vi "optogeneticsTarget3D.vi"(1 "z mode":u16(ring) items=["optogenetics space", "imaging space"], 2 "z device":u16(ring) items=["etl", "piezo"], 3 "xy mode":u16(ring) items=["galvo space", "camera space"], 4 "xyz":dbl[](array[numeric])=[0.0, 0.0, 0.0]) -> ()   [LabVIEW 2017]
uses:
  globalUtilities.vi
  <vilib>/Analysis/NI_AALPro.lvlib
  <vilib>/Analysis/polynomials.llb/Scalar Polynomial Evaluation (DBL).vi
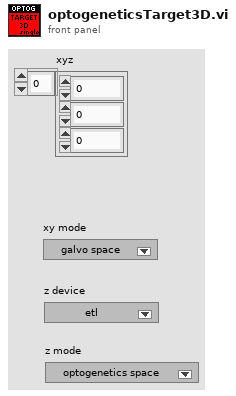
[diagram p1: front panel]
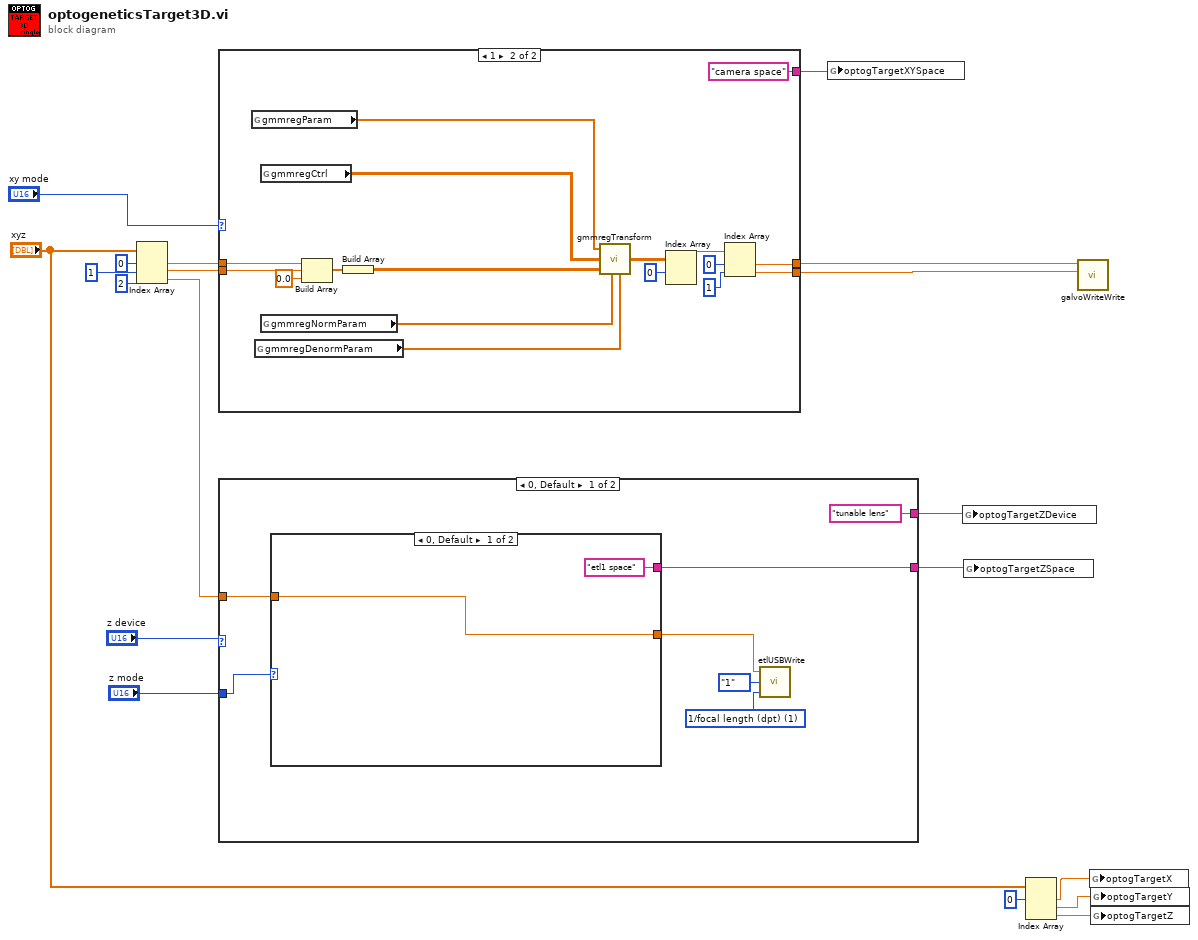
[diagram p0: block diagram]
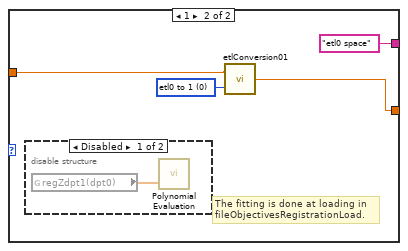
[diagram p2: hidden frame]
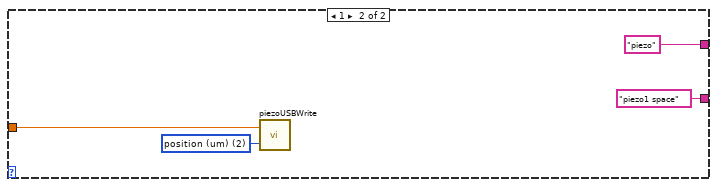
[diagram p4: hidden frame]
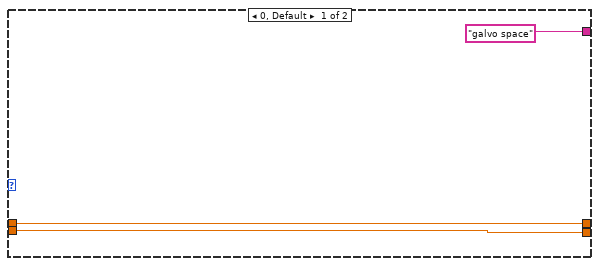
[diagram p5: hidden frame]
diagram:
  n1 = Index Array(array="xyz", index #1=0 ("index"), index #2=1 ("index"), index #3=2 ("index")) -> (element #1=w16:dbl, element #2=w15:dbl, element #3=w10:dbl)
  n2 = case shown="1" "xy mode" {
    tunnel: w16 -> [w22 w36]
    tunnel: w15 -> [w21 w35]
    tunnel: [w22 w26] -> w13
    tunnel: [w21 w25] -> w12
    tunnel: ["galvo space" "camera space"] -> w3
    frame 0, Default {
    }
    frame 1 {
      n3 = global read "globalUtilities.vi" "gmmregParam"() -> (w24:dbl[])
      n4 = global read "globalUtilities.vi" "gmmregDenormParam"() -> (w37:dbl[])
      n5 = global read "globalUtilities.vi" "gmmregCtrl"() -> (w39:dbl[][])
      n6 = global read "globalUtilities.vi" "gmmregNormParam"() -> (w38:dbl[])
      n7 = Build Array(w36, w35, 0.0 ("element")) -> (w33:dbl[])
      n8 = Build Array(w33) -> (w32:dbl[][])
      n9 = call "gmmregTransform.vi"("param0"=w24, "ctrlPts"=w39, "pts"=w32, "normParams"=w38, "denormParams"=w37) -> ("out"=w31:dbl[][])  [unwired: 4 in]
      n10 = Index Array(array=w31, index (row)=0) -> (element=w29:dbl[])  [unwired: 1 in]
      n11 = Index Array(array=w29, index #1=0 ("index"), index #2=1 ("index")) -> (element #1=w26:dbl, element #2=w25:dbl)
    }
  }
  n12 = case shown="0, Default" "z device" {
    tunnel: w10 -> [w45 w57]
    tunnel: "z mode" -> [w46 _]
    tunnel: ["tunable lens" "piezo"] -> w1
    tunnel: [w40 "piezo1 space"] -> w2
    frame 0, Default {
      w43 = u16 1 items=["position (um)", "1/focal length (dpt)"] ("mode")
      n13 = case shown="0, Default" w46 {
        tunnel: w45 -> [w48 w52]
        tunnel: [w48 w50] -> w42
        tunnel: ["etl1 space" "etl0 space"] -> w40
        frame 0, Default {
        }
        frame 1 {
          w51 = u16 0 items=["etl0 to 1", "etl1 to 0"] ("mode")
          # "The fitting is done at loading in\nfileObjectivesRegistrationLoad."
          n14 = disable-structure shown="Disabled" {
            frame Disabled {
              n15 = global read "globalUtilities.vi" "regZdpt1(dpt0)"() -> (w53:dbl[])
              n16 = call-poly <vilib>:"Polynomial Evaluation.vi"("P(x)"=w53) -> ()  [unwired: 1 in, 2 out]
            }
            frame Enabled {
            }
          }
          n17 = call "etlConversion01.vi"("mode"=w51, "in"=w52) -> ("out"=w50:dbl)
        }
      }
      n18 = call "etlUSBWrite.vi"("mode"=w43, "lens"=enum16{"0", "1"}."1", "input"=w42) -> ()  [unwired: 1 in]
    }
    frame 1 {
      w56 = u16 2 items=["fractional", "voltage (V)", "position (um)"] ("mode")
      n19 = call "piezoUSBWrite.vi"("mode"=w56, "position"=w57) -> ()  [unwired: 1 in]
    }
  }
  n20 = global write "globalUtilities.vi" "optogTargetXYSpace"(w3) -> ()
  n21 = global write "globalUtilities.vi" "optogTargetZDevice"(w1) -> ()
  n22 = global write "globalUtilities.vi" "optogTargetZSpace"(w2) -> ()
  n23 = Index Array(array="xyz", index #1=0 ("index")) -> (element #1=w4:dbl, element #2=w5:dbl, element #3=w6:dbl)  [unwired: 2 in]
  n24 = call "galvoWriteWrite.vi"("X"=w13, "Y"=w12) -> ()  [unwired: 4 in]
  n25 = global write "globalUtilities.vi" "optogTargetX"(w4) -> ()
  n26 = global write "globalUtilities.vi" "optogTargetY"(w5) -> ()
  n27 = global write "globalUtilities.vi" "optogTargetZ"(w6) -> ()
